vi "CreateDa.vi"(0 "Sig_DA in":refnum<class "DA.lvclass">, 5 "error in (no error)":errorcluster, 10 "bool_setting":T1, 12 "Tags":T2, 13 "Logger":refnum<class "Logger.lvclass">) -> (14 "Sig_DA out":refnum<class "DA.lvclass">, 19 "error out":errorcluster)   [LabVIEW 2019, in "DA.lvclass"]
uses:
  DA.lvclass
  D:/GIT H4000/H4000/src/Signal_class/Signal.lvclass
  Logger_class/Logger.lvclass
  Proccess_class/TAGs.ctl
  TypeDef/bool_setting.ctl
  DA.lvclass/DA.ctl
  Signal_class/Signal.lvclass
  Proccess_class/Proccess.lvclass
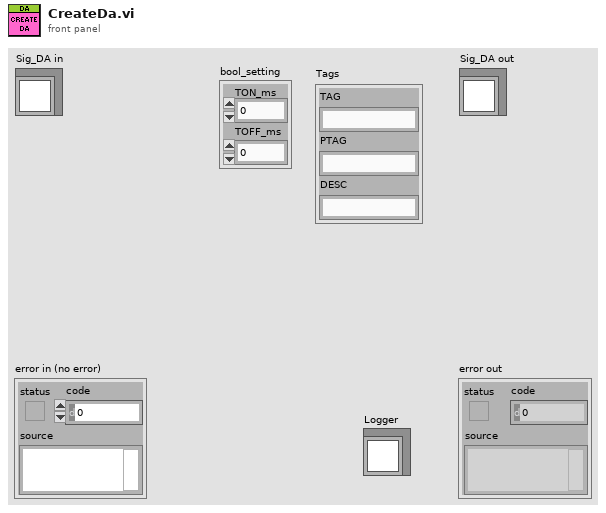
[diagram p1: front panel]
types:
  T1 = typedef "bool_setting.ctl" = cluster{"TON_ms":u32, "TOFF_ms":u32}
  T2 = typedef "Proccess.lvclass/TAGs.ctl" = cluster{"TAG":string, "PTAG":string, "DESC":string}
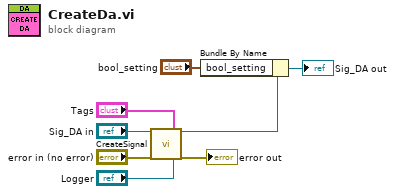
[diagram p0: block diagram]
diagram:
  n1 = call "CreateSignal.vi"("Signal in"="Sig_DA in", "error in (no error)"="error in (no error)", "Tags"="Tags", "Logger"="Logger") -> ("Signal out"=w7:refnum<class "DA.lvclass">, "error out"=→"error out":errorcluster)  [unwired: 14 in]
  n2 = Bundle By Name(cluster=w7, "bool_setting"="bool_setting") -> (→"Sig_DA out":refnum<class "DA.lvclass">)
